vi "Test Print.vi"() -> ()   [LabVIEW 2014, in "Arduino LiquidCrystal Wrapper.lvlib"]
uses:
  Arduino LiquidCrystal Wrapper.lvlib
panel:
  out "Bytes count read":u16
  out "Error Out":errorcluster
  in  "Error In":errorcluster
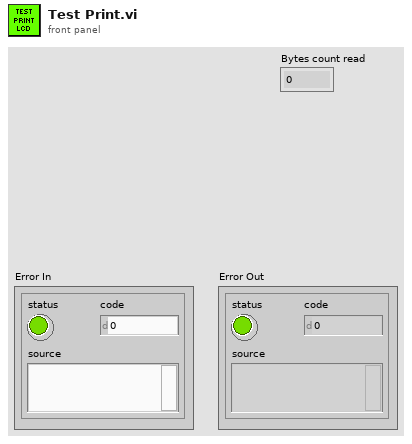
[diagram p1: front panel]
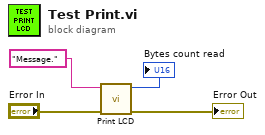
[diagram p0: block diagram]
diagram:
  n1 = call "Print LCD.vi"("Error In"="Error In", "text"="Message.") -> ("Error Out"=→"Error Out":errorcluster, "Bytes count read"=→"Bytes count read":u16)  [unwired: 8 in]
